vi "Voltmeter TSP K2450.vi"(1 "Action":T4=enum."Identify", 2 "Parameters":variant) -> (6 "Output":variant, 7 "Stop":bool)   [LabVIEW 2025]
doc: "This VI reads a single reading from a Keithley 2001 multimeter. The stop boolean is always false. If no reading is obtained a single zero is returned.\nScott Hannahs, NHMFL-FSU, Nov 1993 \nAuthor: Scott Hannahs <sth@magnet.fsu.edu>\n\nThis software is licensed for use under the “MIT License\"\nCopyright (c) 2025 Scott Hannahs, sth@sth@magnet.sthnet.net\n\nPermission is hereby granted, free of charge, to any person obtaining a copy of this software and associated documentation files (the \"Software\"), to deal in the Software without restriction, including without limitation the rights to use, copy, modify, merge, publish, distribute, sublicense, and/or sell copies of the Software, and to permit persons to whom the Software is furnished to do so, subject to the following conditions: The above copyright notice and this permission notice shall be included in all copies or substantial portions of the Software.\n\nTHE SOFTWARE IS PROVIDED \"AS IS\", WITHOUT WARRANTY OF ANY KIND, EXPRESS OR IMPLIED, INCLUDING BUT NOT LIMITED TO THE WARRANTIES OF MERCHANTABILITY, FITNESS FOR A PARTICULAR PURPOSE AND NONINFRINGEMENT. IN NO EVENT SHALL THE AUTHORS OR COPYRIGHT HOLDERS BE LIABLE FOR ANY CLAIM, DAMAGES OR OTHER LIABILITY, WHETHER IN AN ACTION OF CONTRACT, TORT OR OTHERWISE, ARISING FROM, OUT OF OR IN CONNECTION WITH THE SOFTWARE OR THE USE OR OTHER DEALINGS IN THE SOFTWARE."
uses:
  New NML Data Acq/Sub Controls/Instrument Actions.ctl
  New NML Data Acq/Sub Controls/Instrument Match.ctl
  New NML Data Acq/Sub Controls/Public.ctl
  New NML Data Acq/Sub Controls/Factory Reset.ctl
  New NML Data Acq/Sub Controls/Scan Input.ctl
  New NML Data Acq/Sub Controls/Scan Output.ctl
  New NML Data Acq/Sub Controls/Instrument IDN.ctl
  New NML Data Acq/Sub Controls/User Event Command.ctl
panel:
  in  "Factory Reset":T1
  in  "Elements":bool
  in  "Mode Sourcemeter":enum32{"Voltage", "Current", "Both"}(radio)
  out "Title":string
  in  "Public":T2
  in  "Address":u16(ring)
  out "Model":string
  in  "Instruments":T3[](array[typedef])=[{"Model"="34401", "Manufacturer"="HEWLETT-PACKARD", "Term Character"="", "Wait Time (mS)"=0, "Wait for SRQ"=FALSE, "Type"="Voltmeter"}, {"Model"="MODEL 182", "Manufacturer"="KEITHLEY INSTRUMENTS", "Term Character"="", "Wait Time (mS)"=0, "Wait for SRQ"=FALSE, "Type"="Voltmeter"}, {"Model"="MODEL 200[012]", "Manufacturer"="KEITHLEY INSTRUMENTS", "Term Character"="", "Wait Time (mS)"=0, "Wait for SRQ"=FALSE, "Type"="Voltmeter"}, {"Model"="MODEL 6221[A]*", "Manufacturer"="KEITHLEY INSTRUMENTS", "Term Character"="", "Wait Time (mS)"=0, "Wait for SRQ"=FALSE, "Type"="Voltmeter"}, {"Model"="MODEL 2420", "Manufacturer"="KEITHLEY INSTRUMENTS", "Term Character"="", "Wait Time (mS)"=0, "Wait for SRQ"=FALSE, "Type"="Voltmeter"}, {"Model"="MODEL 2182[A]*", "Manufacturer"="KEITHLEY INSTRUMENTS", "Term Character"="", "Wait Time (mS)"=0, "Wait for SRQ"=FALSE, "Type"="Voltmeter"}, {"Model"="MODEL 6517[AB]", "Manufacturer"="KEITHLEY INSTRUMENTS", "Term Character"="", "Wait Time (mS)"=0, "Wait for SRQ"=FALSE, "Type"="Electrometer"}, {"Model"="MODEL 6430", "Manufacturer"="KEITHLEY INSTRUMENTS", "Term Character"="", "Wait Time (mS)"=0, "Wait for SRQ"=FALSE, "Type"="Sourcemeter"}, {"Model"="5313[12]A", "Manufacturer"="HEWLETT-PACKARD", "Term Character"="", "Wait Time (mS)"=0, "Wait for SRQ"=FALSE, "Type"="Counter"}, {"Model"="MODEL 2450", "Manufacturer"="KEITHLEY INSTRUMENTS", "Term Character"="", "Wait Time (mS)"=0, "Wait for SRQ"=FALSE, "Type"="SMU TSP"}, {"Model"="MODEL DMM7510", "Manufacturer"="KEITHLEY INSTRUMENTS", "Term Character"="", "Wait Time (mS)"=0, "Wait for SRQ"=FALSE, "Type"="Voltmeter"}]
  out "Measurement":dbl[](array[numeric]) format="%^_7e"
  in  "VISA resource name":refnum<visa-resource-name>
  # "Term Char"
  # "Wait Time (mS)"
  # "Wait for SRQ?"
  # "Type"
  # "Manufacturer"
  # "Model"
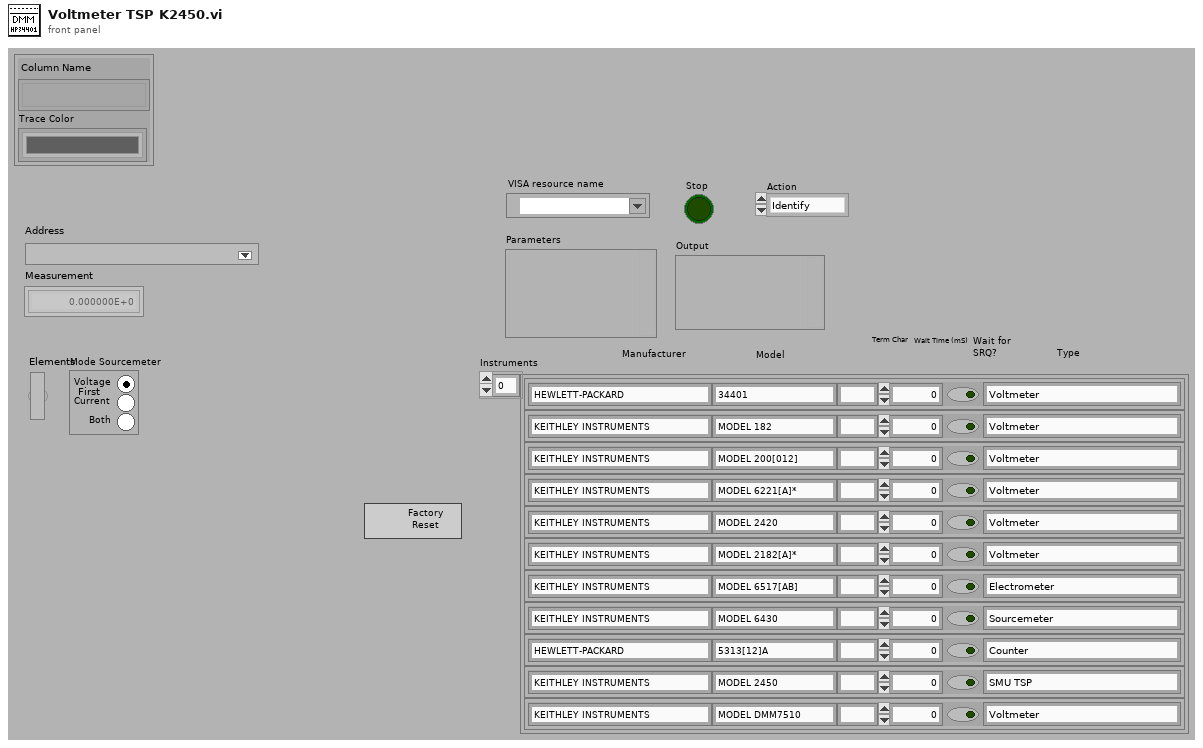
[diagram p1: front panel]
types:
  T1 = typedef "Factory Reset.ctl" = bool
  T2 = typedef "Public.ctl" = cluster{"Column Name":string[], "Trace Color":u32[]}
  T3 = typedef "Instrument Match.ctl" = cluster{"Model":string, "Manufacturer":string, "Term Character":string, "Wait Time (mS)":u32, "Wait for SRQ":bool, "Type":string}
  T4 = typedef "Instrument Actions.ctl" = enum16{"Scan", "Identify", "New", "Configure", "Initialize", "Test", "Read", "Close"}
  T5 = typedef "Scan Output.ctl" = cluster{"Manufacturer":string, "Model":string, "Info":string, "Revision":string, "error out":errorcluster}
  T6 = typedef "Scan Input.ctl" = cluster{"VISA resource name":refnum<visa-resource-name>, "ID String in":string}
  T7 = typedef "Instrument IDN.ctl" = cluster{"VISA Address":string, "Status":u16, "Manufacturer":string, "Model":string, "Info":string, "Info 2":string, "Misc Data":variant}
  T8 = typedef "User Event Command.ctl" = enum32{"Stop Config"}
  T9 = typedef "Instrument Properties.ctl" = cluster{"Public":T2, "Private":T10}
  T10 = typedef "Private.ctl" = cluster{"Path":path, "VI Refnum":T11, "Name":string, "# of Values":i32, "Scale Factors":dbl[], "Display":T12[], "Offset":dbl[]}
  T11 = typedef "Instrument Ref.ctl" = refnum<vi>
  T12 = typedef "SystemCheckBox-resize.ctl" = bool
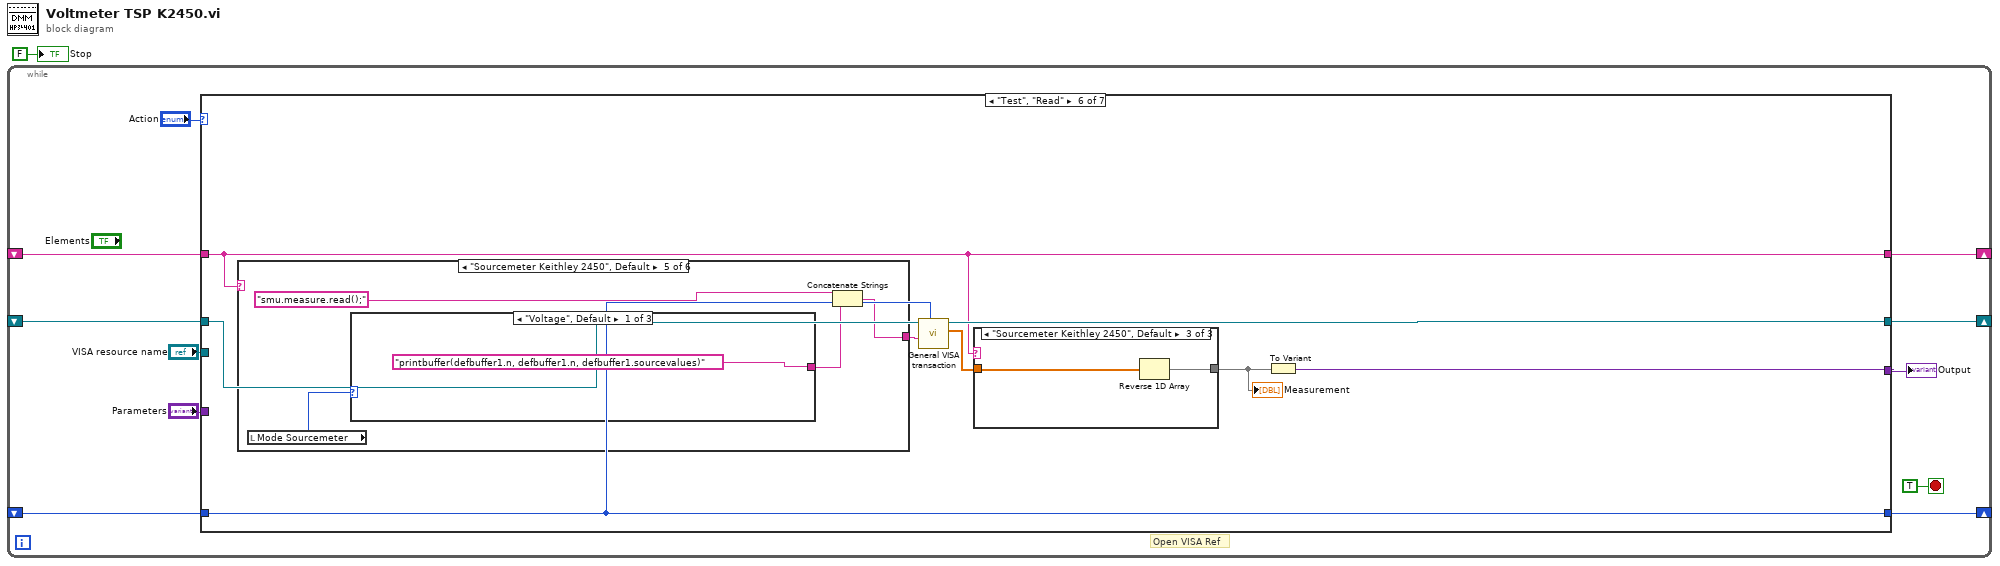
[diagram p0: block diagram]
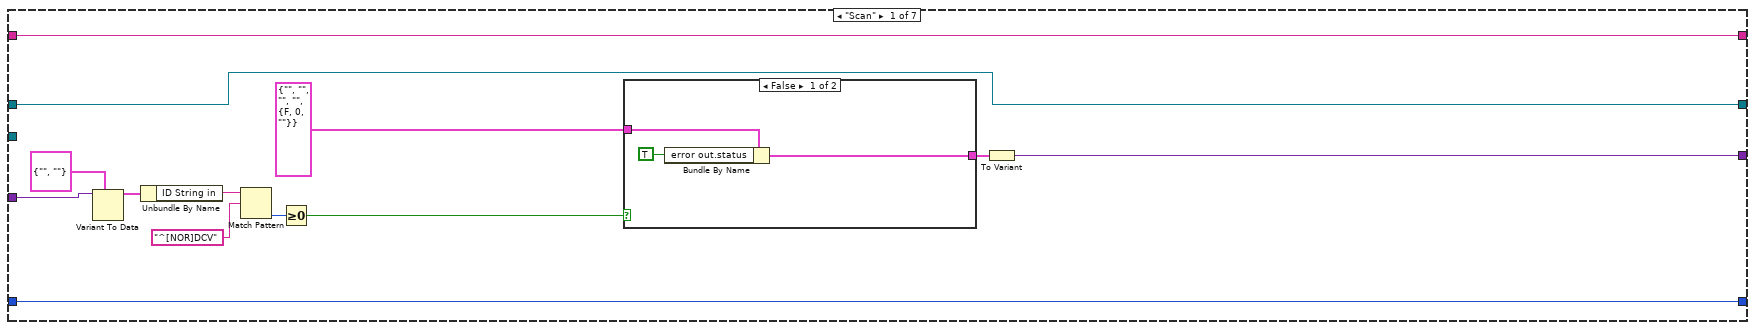
[diagram p2: hidden frame]
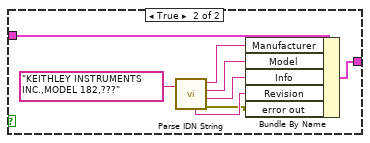
[diagram p3: hidden frame]
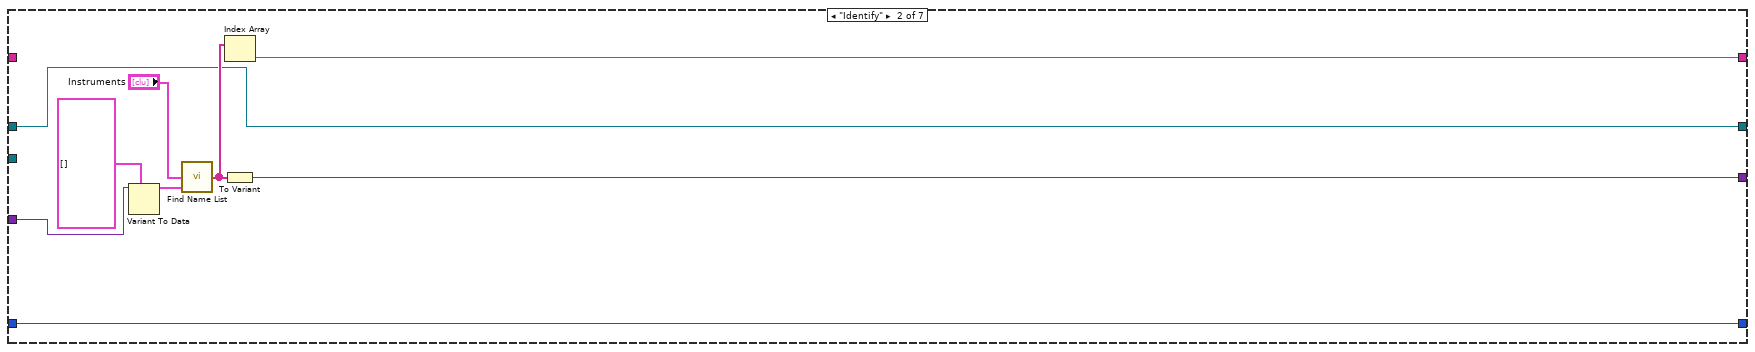
[diagram p4: hidden frame]
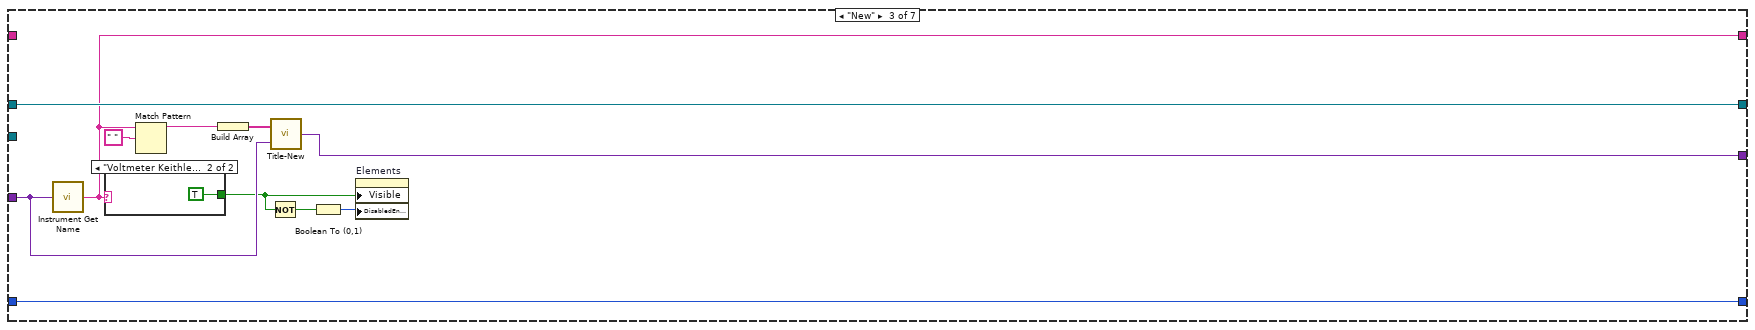
[diagram p5: hidden frame]
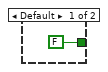
[diagram p6: hidden frame]
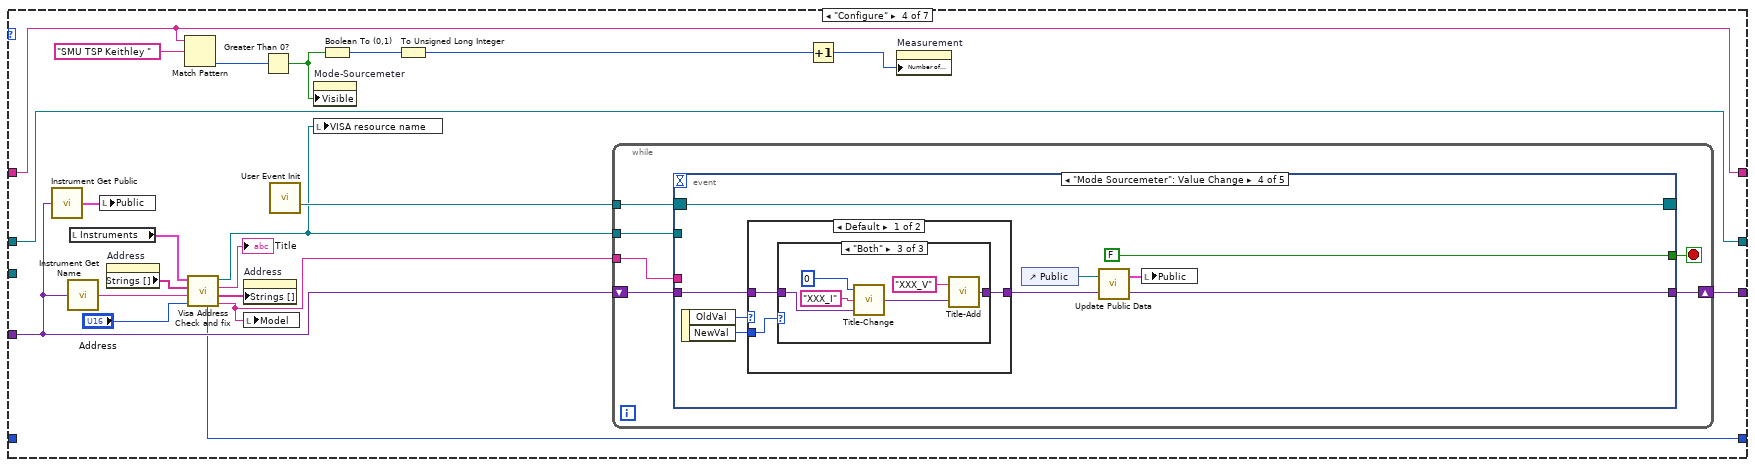
[diagram p7: hidden frame]
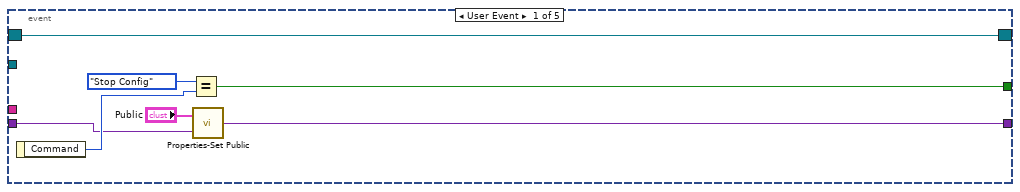
[diagram p8: hidden frame]
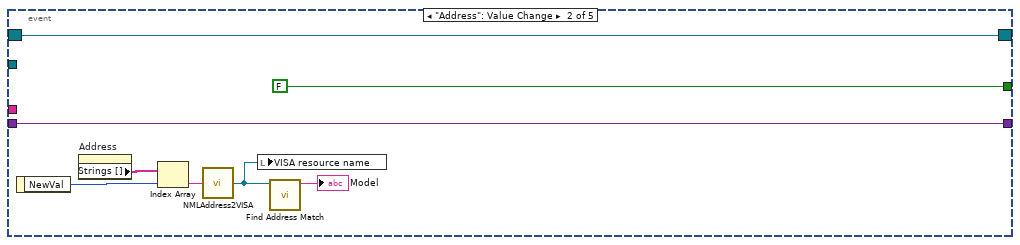
[diagram p9: hidden frame]
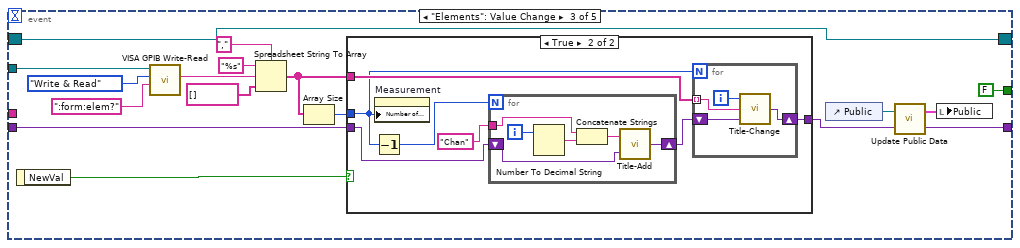
[diagram p10: hidden frame]
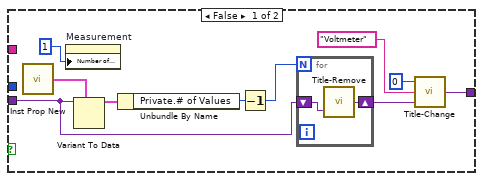
[diagram p11: hidden frame]
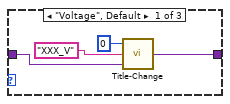
[diagram p12: hidden frame]
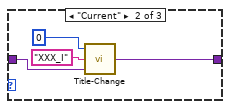
[diagram p13: hidden frame]
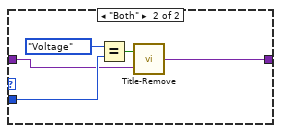
[diagram p14: hidden frame]
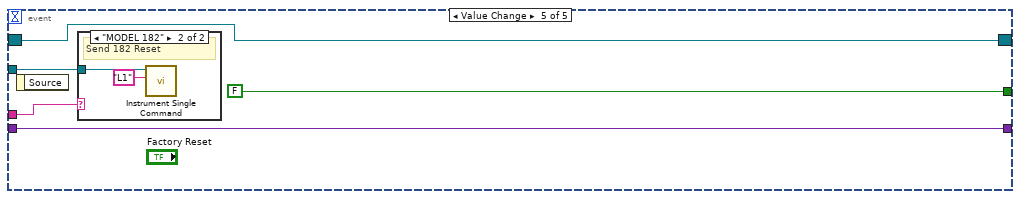
[diagram p15: hidden frame]
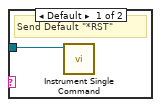
[diagram p16: hidden frame]
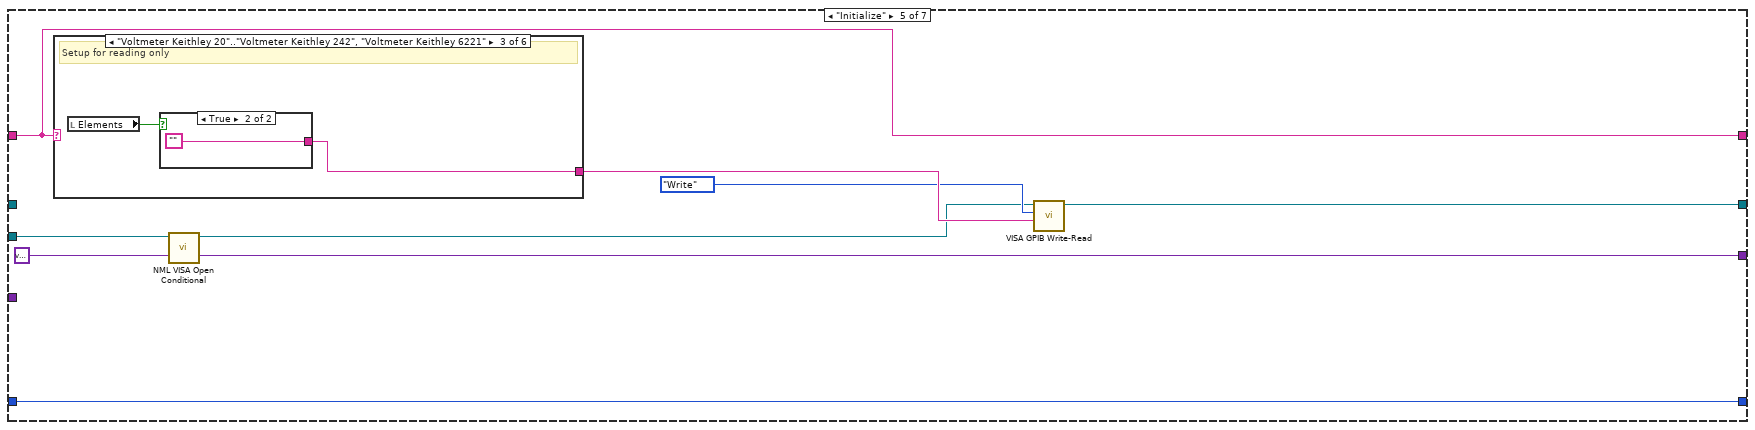
[diagram p17: hidden frame]
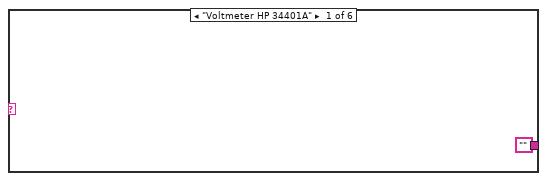
[diagram p18: hidden frame]
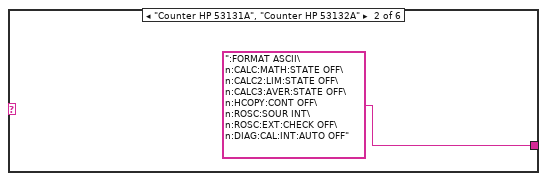
[diagram p19: hidden frame]
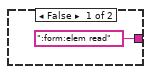
[diagram p20: hidden frame]
diagram:
  n1 = while {
    shift-right: [w8] -> _
    shift-left: _ -> [w7]
    shift-right: [w5] -> _
    shift-left: _ -> [w4]
    shift-right: [w3] -> _
    shift-left: _ -> [w2]
    stop <- TRUE stop-if-true
    # "Open VISA Ref"
    n2 = case shown="\"Test\", \"Read\"" "Action" {
      tunnel: [w18 w45 w56 w74 variant ("Variant") w210 variant ("Variant")] -> w10
      tunnel: "VISA resource name" -> [_ _ _ _ w193 _ _]
      tunnel: [w17 w40 w50 w65 w190 w204 w241] -> w8
      tunnel: w7 -> [w17 _ _ w65 w190 w204 w241]
      tunnel: "Parameters" -> [w25 w44 w54 w71 _ _ _]
      tunnel: [w14 w38 w55 w72 w189 w208 refnum<visa-resource-name> refnum ("Open VISA Resource name")] -> w5
      tunnel: w4 -> [w14 w38 w55 w72 _ w209 w239]
      tunnel: [w13 w37 w46 w59 w186 w203 w238] -> w3
      tunnel: w2 -> [w13 w37 w46 _ w186 w203 w238]
      frame "Scan" {
        n3 = Variant To Data(type=T6 {"VISA resource name"="", "ID String in"=""} ("Scan Input"), Variant=w25) -> (data=w23:T6)  [unwired: 1 in, 1 out]
        n4 = Unbundle By Name(w23) -> ("ID String in"=w20:string)
        n5 = Match Pattern(string=w20, regular expression="^[NOR]DCV") -> (offset past match=w22:i32)  [unwired: 1 in, 3 out]
        n6 = Greater Or Equal To 0?(x=w22) -> (x >= 0?=w19:bool)
        n7 = case shown="False" w19 {
          tunnel: T5 {"Manufacturer"="", "Model"="", "Info"="", "Revision"="", "error out"={"status"=FALSE, "code"=0, "source"=""}} ("Scan Output") -> [w27 w36]
          tunnel: [w28 w35] -> w15
          frame False {
            n8 = Bundle By Name(cluster=w27, "error out.status"=TRUE) -> (w28:T5)
          }
          frame True {
            n9 = call "Parse IDN String.vi"("IDN String"="KEITHLEY INSTRUMENTS INC.,MODEL 182,???") -> ("error out"=w32:errorcluster, "Info"=w31:string, "Model"=w30:string, "Manufacturer"=w29:string, "Revision"=w33:string)  [unwired: 1 in]
            n10 = Bundle By Name(cluster=w36, "Manufacturer"=w29, "Model"=w30, "Info"=w31, "Revision"=w33, "error out"=w32) -> (w35:T5)
          }
        }
        n11 = To Variant(anything=w15) -> (Variant=w18:variant)
      }
      frame "Identify" {
        n12 = Variant To Data(type=T7[] [], Variant=w44) -> (data=w42:T7[])  [unwired: 1 in, 1 out]
        n13 = call "Find Name List.vi"("Bus Scan"=w42, "Instruments"="Instruments") -> ("Names"=w39:string[])  [unwired: 1 in]
        n14 = Index Array(array=w39) -> (element=w40:string)  [unwired: 1 in]
        n15 = To Variant(anything=w39) -> (Variant=w45:variant)
      }
      frame "New" {
        n16 = call "Instrument Get Name.vi"("Parameters"=w54) -> ("Type"=w50:string)
        n17 = case shown="\"Voltmeter Keithley 6221\"" w50 {
          tunnel: [FALSE ("Visible") TRUE ("Visible")] -> w49
          frame Default {
          }
          frame "Voltmeter Keithley 6221" {
          }
        }
        n18 = Match Pattern(string=w50, regular expression=" ") -> (before substring=w52:string)  [unwired: 1 in, 3 out]
        n19 = Build Array(w52) -> (w53:string[])
        n20 = Not(x=w49) -> (.not. x?=w47:bool)
        n21 = call "Title-New.vi"("Parameters"=w54, "Array"=w53) -> ("Instrument Prop"=w56:variant)
        n22 = Boolean To (0,1)(Boolean=w47) -> (0, 1=w48:i16)
        n23 = property on="Elements" class="Bool (strict)"("Visible"=w49, "DisabledEnum"=w48) -> ()  [unwired: 2 in, 2 out]
      }
      frame "Configure" {
        n24 = call "Instrument Get Public.vi"("Variant"=w71) -> ("Public"=w75:T2)
        n25 = call "Instrument Get Name.vi"("Parameters"=w71) -> ("Type"=w70:string)
        n26 = local read "Instruments"() -> (w76:T3[])
        n27 = local write "Public"(w75) -> ()
        n28 = property on="Address" class="Ring (strict)"() -> ("Strings []"=w77:string[])  [unwired: 2 in, 2 out]
        n29 = Match Pattern(string=w65, regular expression="SMU TSP Keithley " ("y")) -> (offset past match=w63:i32)  [unwired: 1 in, 3 out]
        n30 = call "Visa Address Check and fix.vi"("Instruments"=w76, "NML Addresses"=w77, "Name"=w70, "Address"="Address") -> ("Wait Time (mS)"=w59:u32, "VISA resource name"=w61:refnum<visa-resource-name>, "Title"=→"Title":string, "NML Addresses"=w79:string[], "Model"=w60:string)  [unwired: 2 out]
        n31 = property on="Address" class="Ring (strict)"("Strings []"=w79) -> ()  [unwired: 2 in, 2 out]
        n32 = local write "Model"(w60) -> ()
        n33 = Greater Than 0?(x=w63) -> (x > 0?=w62:bool)
        n34 = call "User Event Init.vi"() -> ("Event Registration Refnum"=w73:refnum<event-registration>)  [unwired: 14 in, 1 out]
        n35 = property on="Mode-Sourcemeter" class="RadioBtnsControl (strict)"("Visible"=w62) -> ()  [unwired: 2 in, 2 out]
        n36 = local write "VISA resource name"(w61) -> ()
        n37 = Boolean To (0,1)(Boolean=w62) -> (0, 1=w68:i16)
        n38 = To Unsigned Long Integer(number=w68) -> (unsigned 32bit integer=w66:u32)
        n39 = while {
          tunnel: w73 -> [w82]
          shift-right: [w85] -> w74
          shift-left: w71 -> [w83]
          tunnel: w61 -> [w81]
          tunnel: w60 -> [w80]
          stop <- w84 stop-if-true
          n40 = event shown="[3] \"Mode Sourcemeter\": Value Change" {
            selector: w82 -> [w86 w94 w114 w155 w178]
            dyn-events: [w86 w94 w114 w155 w178] -> _
            timeout: _ -> [_ _ _ _ _]
            tunnel: [w90 w95 w111 w149 w180] -> w85
            tunnel: [w88 FALSE FALSE FALSE FALSE] -> w84
            tunnel: w83 -> [w91 w95 w117 w151 w180]
            tunnel: w81 -> [_ _ w107 _ w182]
            tunnel: w80 -> [_ _ _ _ w181]
            event User Event {
              n41 = event-data() -> ("Command"=w92:T8)  [unwired: 1 in]
              n42 = Equal?(x=User_Event_Command."Stop Config", y=w92) -> (x = y?=w88:bool)
              n43 = call "Properties-Set Public.vi"("Variant"=w91, "New Public"="Public") -> ("Variant 2"=w90:variant)
            }
            event "Address": Value Change {
              n44 = event-data() -> ("NewVal"=w100:u16)  [unwired: 1 in]
              n45 = property on="Address" class="Ring (strict)"() -> ("Strings []"=w97:string[])  [unwired: 2 in, 2 out]
              n46 = Index Array(array=w97, index=w100) -> (element=w98:string)
              n47 = call "NMLAddress2VISA.vi"("NML Address"=w98) -> ("VISA resource name"=w93:refnum<visa-resource-name>)
              n48 = local write "VISA resource name"(w93) -> ()
              n49 = call "Find Address Match.vi"("VISA resource name"=w93) -> ("Model"=→"Model":string)  [unwired: 3 in, 3 out]
            }
            event "Elements": Value Change {
              n50 = event-data() -> ("NewVal"=w116:bool)  [unwired: 1 in]
              n51 = call "VISA GPIB Write-Read.vi"("Command"=":form:elem?", "Action"=enum16{"Write", "Read", "Write & Read"}."Write & Read", "VISA resource name"=w107) -> ("String Returned"=w106:string)  [unwired: 5 in, 3 out]
              n52 = Spreadsheet String To Array(delimiter (Tab)=",", format string="%s", spreadsheet string=w106, array type (2D Dbl)=string[] [] ("array")) -> (array=w101:string[])
              n53 = Array Size(array=w101) -> (size(s)=w103:i32)
              n54 = case shown="True" w116 {
                tunnel: w117 -> [w124 w135]
                tunnel: [w121 w131] -> w112
                tunnel: w103 -> [_ w132]
                tunnel: w101 -> [_ w133]
                frame False {
                  n55 = call "Inst Prop New.vi"() -> ("Instrument Prop Out"=w127:T9)
                  n56 = property on="Measurement" class="Arr (strict)"("Number of Columns"=u32 1) -> ()  [unwired: 2 in, 2 out]
                  n57 = Variant To Data(type=w127, Variant=w124) -> (data=w126:T9)  [unwired: 1 in, 1 out]
                  n58 = Unbundle By Name(w126) -> ("Private.# of Values"=w125:i32)
                  n59 = Decrement(x=w125) -> (x-1=w119:i32)
                  n60 = for {
                    N: w119 -> [_]
                    shift-right: [w129] -> w122
                    shift-left: w124 -> [w128]
                    n61 = call "Title-Remove.vi"("Parameters"=w128) -> ("Variant"=w129:variant)  [unwired: 1 in]
                  }
                  n62 = call "Title-Change.vi"("Parameters"=w122, "New Title"="Voltmeter", "Index"=0) -> ("Variant"=w121:variant)
                }
                frame True {
                  n63 = Decrement(x=w132) -> (x-1=w136:i32)
                  n64 = property on="Measurement" class="Arr (strict)"("Number of Columns"=w132) -> ()  [unwired: 2 in, 2 out]
                  n65 = for {
                    N: w136 -> [_]
                    tunnel: "Chan" ("String") -> [w145]
                    shift-right: [w146] -> w130
                    shift-left: w135 -> [w141]
                    i -> [w143]
                    n66 = Number To Decimal String(number=w143) -> (decimal integer string=w142:string)  [unwired: 1 in]
                    n67 = Concatenate Strings(w145, w142) -> (w144:string)
                    n68 = call "Title-Add.vi"("Parameters"=w141, "String"=w144) -> ("Variant"=w146:variant)
                  }
                  n69 = for {
                    N: w132 -> [_]
                    tunnel: w133 -> [w139] mode=indexing
                    shift-right: [w138] -> w131
                    shift-left: w130 -> [w137]
                    i -> [w140]
                    n70 = call "Title-Change.vi"("Parameters"=w137, "New Title"=w139, "Index"=w140) -> ("Variant"=w138:variant)
                  }
                }
              }
              n71 = control-ref of="Public"() -> (w110:refnum<vi>)
              n72 = call "Update Public Data.vi"("Variant In"=w112, "Public 2"=w110) -> ("Variant Out"=w111:variant, "Public"=w113:T2)
              n73 = local write "Public"(w113) -> ()
            }
            event "Mode Sourcemeter": Value Change {
              n74 = event-data() -> ("OldVal"=w153:enum32{"Voltage", "Current", "Both"}, "NewVal"=w152:enum32{"Voltage", "Current", "Both"})  [unwired: 1 in]
              n75 = case shown="Default" w153 {
                tunnel: w152 -> [w158 w176]
                tunnel: w151 -> [w157 w173]
                tunnel: [w156 w177] -> w150
                frame Default {
                  n76 = case shown="\"Both\"" w158 {
                    tunnel: w157 -> [w162 w163 w170]
                    tunnel: [w159 w164 w168] -> w156
                    frame "Voltage", Default {
                      n77 = call "Title-Change.vi"("Parameters"=w162, "New Title"="XXX_V", "Index"=0) -> ("Variant"=w159:variant)
                    }
                    frame "Current" {
                      n78 = call "Title-Change.vi"("Parameters"=w163, "New Title"="XXX_I", "Index"=0) -> ("Variant"=w164:variant)
                    }
                    frame "Both" {
                      n79 = call "Title-Change.vi"("Parameters"=w170, "New Title"="XXX_I", "Index"=0) -> ("Variant"=w169:variant)
                      n80 = call "Title-Add.vi"("Parameters"=w169, "String"="XXX_V") -> ("Variant"=w168:variant)
                    }
                  }
                }
                frame "Both" {
                  n81 = Equal?(x=enum32{"Voltage", "Current", "Both"}."Voltage", y=w176) -> (x = y?=w174:bool)
                  n82 = call "Title-Remove.vi"("Parameters"=w173, "Remove First"=w174) -> ("Variant"=w177:variant)
                }
              }
              n83 = control-ref of="Public"() -> (w147:refnum<vi>)
              n84 = call "Update Public Data.vi"("Variant In"=w150, "Public 2"=w147) -> ("Variant Out"=w149:variant, "Public"=w148:T2)
              n85 = local write "Public"(w148) -> ()
            }
            event Value Change {
              n86 = event-data() -> ()  [unwired: 1 in, 1 out]
              n87 = case shown="\"MODEL 182\"" w181 {
                tunnel: w182 -> [w183 w185]
                frame Default {
                  # "Send Default \"*RST\""
                  n88 = call "Instrument Single Command.vi"("VISA Name"=w183) -> ()  [unwired: 10 in, 1 out]
                }
                frame "MODEL 182" {
                  # "Send 182 Reset"
                  n89 = call "Instrument Single Command.vi"("Reset Command"="L1", "VISA Name"=w185) -> ()  [unwired: 9 in, 1 out]
                }
              }
            }
          }
        }
        n90 = Increment(x=w66) -> (x+1=w67:u32)
        n91 = property on="Measurement" class="Arr (strict)"("Number of Columns"=w67) -> ()  [unwired: 2 in, 2 out]
      }
      frame "Initialize" {
        n92 = case shown="\"Voltmeter Keithley 20\"..\"Voltmeter Keithley 242\", \"Voltmeter Keithley 6221\"" w190 {
          tunnel: ["" ":FORMAT ASCII\n:CALC:MATH:STATE OFF\n:CALC2:LIM:STATE OFF\n:CALC3:AVER:STATE OFF\n:HCOPY:CONT OFF\n:ROSC:SOUR INT\n:ROSC:EXT:CHECK OFF\n:DIAG:CAL:INT:AUTO OFF" w197 ":form:elem VOLT,CURR" "" ""] -> w191
          frame "Voltmeter HP 34401A" {
          }
          frame "Counter HP 53131A", "Counter HP 53132A" {
          }
          frame "Voltmeter Keithley 20".."Voltmeter Keithley 242", "Voltmeter Keithley 6221" {
            # "Setup for reading only"
            n93 = local read "Elements"() -> (w196:bool)
            n94 = case shown="True" w196 {
              tunnel: [":form:elem read" ""] -> w197
              frame False {
              }
              frame True {
              }
            }
          }
          frame "Sourcemeter Keithley 6430" {
          }
          frame "Electrometer Keithley 6517A", "Electrometer Keithley 6517B" {
          }
          frame "Voltmeter Keithley 182", Default {
          }
        }
        n95 = call "NML VISA Open Conditional.vi"("VISA resource name"=w193) -> ("dup VISA Session"=w187:refnum<visa-resource-name>)  [unwired: 8 in, 2 out]
        n96 = call "VISA GPIB Write-Read.vi"("Command"=w191, "Action"=enum16{"Write", "Read", "Write & Read"}."Write", "VISA resource name"=w187) -> ("dup VISA Session"=w189:refnum<visa-resource-name>)  [unwired: 5 in, 3 out]
      }
      frame "Test", "Read" {
        n97 = case shown="\"Sourcemeter Keithley 2450\", Default" w204 {
          tunnel: ["read?" "fetc?" "Sens:data:latest?" w222 w230 ""] -> w207
          frame "Voltmeter HP 34401A", "Voltmeter Keithley DMM7510" {
          }
          frame "Counter HP 53131A", "Counter HP 53132A" {
          }
          frame "Electrometer Keithley 6517A", "Electrometer Keithley 6517B", "Voltmeter Keithley 2".."Voltmeter Keithley 25", "Voltmeter Keithley 6221" {
          }
          frame "Sourcemeter Keithley 6430" {
            n98 = Not Equal?(x="Mode Sourcemeter", y=enum32{"Voltage", "Current", "Both"}."Current") -> (x != y?=w226:bool)
            n99 = Select(t=":meas:volt?", s=w226, f="") -> (s? t:f=w224:string)
            n100 = Concatenate Strings(":meas:curr?;", w224) -> (w222:string)
          }
          frame "Sourcemeter Keithley 2450", Default {
            n101 = local read "Mode Sourcemeter"() -> (w233:enum32{"Voltage", "Current", "Both"})
            n102 = case shown="\"Voltage\", Default" w233 {
              tunnel: ["printbuffer(defbuffer1.n, defbuffer1.n, defbuffer1.sourcevalues)" "printbuffer(defbuffer1.n, defbuffer1.n, defbuffer1)" "printbuffer(defbuffer1.n, defbuffer1.n, defbuffer1.sourcevalues, defbuffer1.readings)"] -> w231
              frame "Voltage", Default {
              }
              frame "Current" {
              }
              frame "Both" {
              }
            }
            n103 = Concatenate Strings("smu.measure.read();", w231) -> (w230:string)
          }
          frame "Voltmeter Keithley 182" {
          }
        }
        n104 = call "General VISA transaction.vi"("Wait (mS)"=w203, "Command String"=w207, "VISA Session"=w209) -> ("Measurement"=w206:dbl[], "dup VISA Session"=w208:refnum<visa-resource-name>)  [unwired: 3 in, 4 out]
        n105 = case shown="\"Sourcemeter Keithley 2450\", Default" w204 {
          tunnel: [w211 w215 w218] -> w205
          tunnel: w206 -> [w211 w216 w217]
          frame "Test" {
          }
          frame "Sourcemeter Keithley 6430" {
            n106 = Index Array(array=w216, index #1=0 ("index")) -> (element #2=w214:dbl, element #3=w213:dbl)  [unwired: 3 in, 2 out]
            n107 = Build Array(w214, w213) -> (w215:dbl[])
          }
          frame "Sourcemeter Keithley 2450", Default {
            n108 = Reverse 1D Array(array=w217) -> (reversed array=w218:dbl[])
          }
        }
        "Measurement" <- w205
        n109 = To Variant(anything=w205) -> (Variant=w210:variant)
      }
      frame "Close" {
        n110 = call "NML VISA Close.vi"("VISA resource name"=w239) -> ()  [unwired: 10 in, 1 out]
      }
    }
    "Output" <- w10
  }
  "Stop" <- FALSE ("Stop")
